vi "sub_main_imu.vi"(8 "error in":errorcluster) -> (0 "error out":errorcluster)   [LabVIEW 2019]
uses:
  Ctrl/gps-databuf.ctl
panel:
  out "n1":i32
  out "n":i32
  out "n2":i32
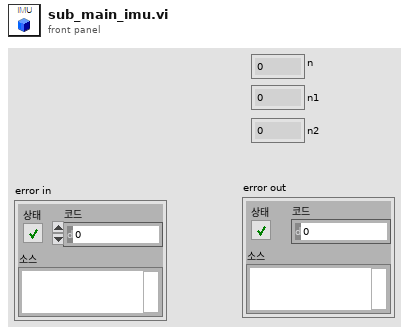
[diagram p1: front panel]
types:
  T1 = typedef "gps-databuf.ctl" = enum16{"read", "write"}
  T2 = typedef "imu-cfg.ctl" = cluster{"Port":refnum<visa-resource-name>, "offset":dbl, "rate":u32}
  T3 = cluster{"rawdata":string, "GPS Data":cluster{"Latitude":cluster{"Valid?":bool, "Latitude (Deg)":dbl}, "Longitude":cluster{"Valid?":bool, "Longitude (Deg)":dbl}, "Height":cluster{"Valid?":bool, "Height (m)":dbl}, "Undulation":cluster{"Valid?":bool, "Undulation(m)":dbl}, "North Vel":cluster{"Valid?":bool, "North Vel (m/s)":dbl}, "East Vel":cluster{"Valid?":bool, "East Vel (m/s)":dbl}, "Up Vel":cluster{"Valid?":bool, "Up Vel (m/s)":dbl}, "Roll":cluster{"Valid?":bool, "Roll (degrees)":dbl}, "Pitch":cluster{"Valid?":bool, "Pitch (degrees)":dbl}, "Azimuth":cluster{"Valid?":bool, "Azimuth (degrees)":dbl}, "Lat deviation":cluster{"Valid?":bool, "Lat deviation (m)":dbl}, "Long deviation":cluster{"Valid?":bool, "Long deviation (m)":dbl}, "Height deviation":cluster{"Valid?":bool, "Height deviation (m)":dbl}, "North vel deviation":cluster{"Valid?":bool, "North vel deviation (m/s)":dbl}, "East vel deviation":cluster{"Valid?":bool, "East vel deviation (m/s)":dbl}, "Up vel deviation":cluster{"Valid?":bool, "Up vel deviation (m/s)":dbl}, "Roll deviation":cluster{"Valid?":bool, "Roll deviation (degrees)":dbl}, "Pitch deviation":cluster{"Valid?":bool, "Pitch deviation (degrees)":dbl}, "Azimuth deviation":cluster{"Valid?":bool, "Azimuth deviation (degrees)":dbl}, "Ext sol status":cluster{"Valid?":bool, "Ext sol status":dbl}}, "Heading":dbl, "utm-1":cluster{"XN":dbl, "YE":dbl}}
  T4 = typedef "error_cluster.ctl" = cluster{"AGV":u8, "AGV Estop":u8, "Obstacle":u8, "Heading":u8, "Waypt":u8, "GNSS":u8, "VLP16":u8, "Cam":u8, "RPLidar":u8, "Joystick":u8, "IMU":u8}
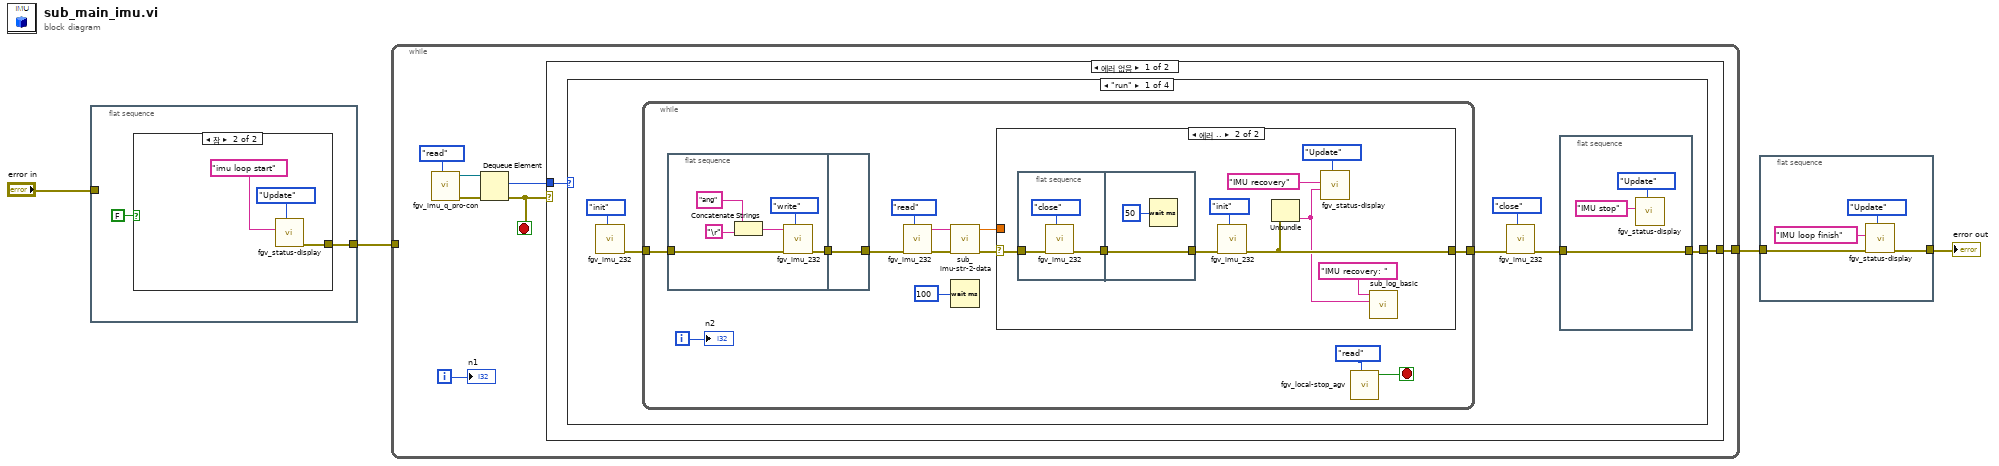
[diagram p0: block diagram]
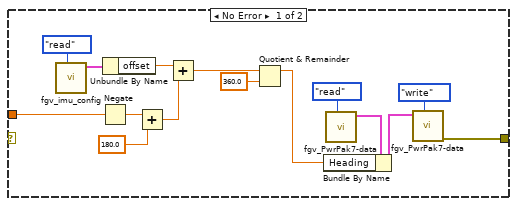
[diagram p2: hidden frame]
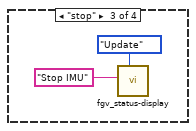
[diagram p4: hidden frame]
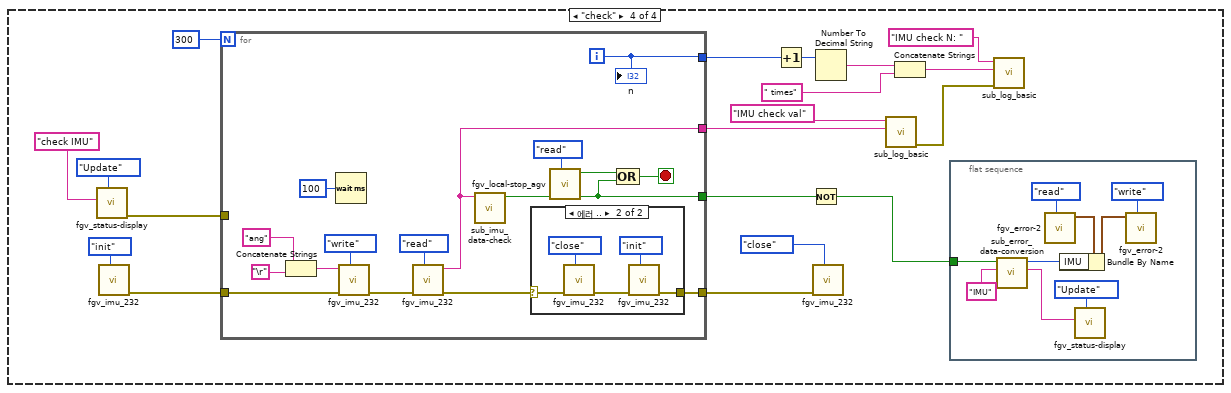
[diagram p5: hidden frame]
diagram:
  n1 = flat-sequence {
    tunnel: [w6] -> w3
    tunnel: "error in" -> [_]
    frame #0 {
      n2 = case shown="참" FALSE {
        tunnel: [_ w7] -> w6
        frame False {
        }
        frame True {
          n3 = call "fgv_status-display.vi"("Mode"=enum16{"Initial", "Update", "Clear"}."Update", "title"="imu loop start" ("String in 1")) -> ("error out"=w7:errorcluster)  [unwired: 9 in]
        }
      }
    }
  }
  n4 = while {
    tunnel: [w15] -> w1
    tunnel: w3 -> [_]
    i -> [w14]
    stop <- w13 stop-if-true
    n5 = call "fgv_imu_q_pro-con.vi"("cmd"=enum16{"create", "write", "read", "close"}."read") -> ("error out"=w10:errorcluster, "queue out"=w11:refnum<queue>)  [unwired: 9 in]
    n6 = Dequeue Element(queue=w11, error in (no error)=w10) -> (element=w16:enum16{"run", "check", "stop"}, error out=w13:errorcluster)  [unwired: 1 in, 2 out]
    n7 = case shown="에러 없음" w13 {
      tunnel: w16 -> [w18 _]
      tunnel: [w17 _] -> w15
      frame No Error {
        n8 = case shown="\"run\"" w18 {
          tunnel: [w24 _ _ _] -> w17
          frame "run" {
            n9 = call "fgv_imu_232.vi"("cmd"=enum16{"init", "read", "write", "close"}."init") -> ("error out"=w22:errorcluster)  [unwired: 8 in, 2 out]
            n10 = while {
              tunnel: [w37] -> w20
              tunnel: w22 -> [w35]
              i -> [w36]
              stop <- w39 stop-if-true
              n11 = flat-sequence {
                tunnel: w35 -> [w42]
                tunnel: [w41] -> w30
                tunnel: [w47] -> w34
                tunnel: w30 -> [w47]
                frame #0 {
                  n12 = Concatenate Strings("ang" ("문자열"), "\r") -> (w46:string)
                  n13 = call "fgv_imu_232.vi"("cmd"=enum16{"init", "read", "write", "close"}."write", "error in"=w42, "write buff"=w46) -> ("error out"=w41:errorcluster)  [unwired: 6 in, 2 out]
                }
                frame #1 {
                }
              }
              n14 = call "fgv_imu_232.vi"("cmd"=enum16{"init", "read", "write", "close"}."read", "error in"=w34) -> ("error out"=w32:errorcluster, "read_buffer"=w33:string)  [unwired: 7 in, 1 out]
              n15 = call "sub_imu-str-2-data.vi"("error in"=w32, "read buffer"=w33) -> ("error out"=w31:errorcluster, "yaw"=w29:dbl)  [unwired: 8 in]
              n16 = Wait (ms)(milliseconds to wait=u32 100 ("대기 시간 (ms)")) -> ()  [unwired: 1 out]
              n17 = case shown="에러 .." w31 {
                selector: w31 -> [_ w71]
                tunnel: [w57 w66] -> w37
                tunnel: w29 -> [w56 _]
                frame No Error {
                  n18 = call "fgv_imu_config.vi"("cmd"=enum16{"read", "write"}."read") -> ("IMU cfg out"=w53:T2)  [unwired: 9 in, 1 out]
                  n19 = Negate(x=w56) -> (-x=w55:dbl)
                  n20 = Unbundle By Name(w53) -> ("offset"=w52:dbl)
                  n21 = Add(x=w55, y=180.0) -> (x+y=w51:dbl)
                  n22 = Add(x=w52, y=w51) -> (x+y=w50:dbl)
                  n23 = Quotient & Remainder(x=w50, y=360.0) -> (x-y*floor(x/y)=w48:dbl)  [unwired: 1 out]
                  n24 = call "fgv_PwrPak7-data.vi"("cmd"=gps-databuf."read") -> ("data cluster out"=w59:T3)  [unwired: 9 in, 1 out]
                  n25 = Bundle By Name(cluster=w59, "Heading"=w48) -> (w60:T3)
                  n26 = call "fgv_PwrPak7-data.vi"("cmd"=gps-databuf."write", "data cluster in"=w60) -> ("error out"=w57:errorcluster)  [unwired: 8 in, 1 out]
                }
                frame Error {
                  n27 = flat-sequence {
                    tunnel: w71 -> [w73]
                    tunnel: [w72] -> w65
                    tunnel: [w76] -> w67
                    tunnel: w65 -> [w76]
                    frame #0 {
                      n28 = call "fgv_imu_232.vi"("cmd"=enum16{"init", "read", "write", "close"}."close", "error in"=w73) -> ("error out"=w72:errorcluster)  [unwired: 7 in, 2 out]
                    }
                    frame #1 {
                      n29 = Wait (ms)(milliseconds to wait=u32 50 ("대기 시간 (ms)")) -> ()  [unwired: 1 out]
                    }
                  }
                  n30 = call "fgv_imu_232.vi"("cmd"=enum16{"init", "read", "write", "close"}."init", "error in"=w67) -> ("error out"=w66:errorcluster)  [unwired: 7 in, 2 out]
                  n31 = Unbundle(w66) -> ("source"=w63:string)  [unwired: 2 out]
                  n32 = call "fgv_status-display.vi"("Mode"=enum16{"Initial", "Update", "Clear"}."Update", "detail"=w63, "title"="IMU recovery" ("String in 1")) -> ()  [unwired: 8 in, 1 out]
                  n33 = call "sub_log_basic.vi"("desc"=w63, "Title"="IMU recovery: ") -> ()  [unwired: 9 in, 1 out]
                }
              }
              n34 = call "fgv_local-stop_agv.vi"("cmd"=enum16{"ini", "read", "stop"}."read") -> ("stop status"=w39:bool)  [unwired: 10 in]
              "n2" <- w36
            }
            n35 = call "fgv_imu_232.vi"("cmd"=enum16{"init", "read", "write", "close"}."close", "error in"=w20) -> ("error out"=w19:errorcluster)  [unwired: 7 in, 2 out]
            n36 = flat-sequence {
              tunnel: [w25] -> w24
              tunnel: w19 -> [w25]
              frame #0 {
                n37 = call "fgv_status-display.vi"("Mode"=enum16{"Initial", "Update", "Clear"}."Update", "title"="IMU stop" ("String in 1")) -> ()  [unwired: 9 in, 1 out]
              }
            }
          }
          frame Default {
          }
          frame "stop" {
            n38 = call "fgv_status-display.vi"("Mode"=enum16{"Initial", "Update", "Clear"}."Update", "title"="Stop IMU" ("String in")) -> ()  [unwired: 9 in, 1 out]
          }
          frame "check" {
            n39 = call "fgv_status-display.vi"("Mode"=enum16{"Initial", "Update", "Clear"}."Update", "title"="check IMU" ("String in")) -> ("error out"=w79:errorcluster)  [unwired: 9 in]
            n40 = call "fgv_imu_232.vi"("cmd"=enum16{"init", "read", "write", "close"}."init") -> ("error out"=w93:errorcluster)  [unwired: 8 in, 2 out]
            n41 = for {
              N: 300 -> [_]
              tunnel: w93 -> [w113]
              tunnel: [w115] -> w91
              tunnel: [w107] -> w90
              tunnel: [w117] -> w86
              tunnel: [w108] -> w85
              tunnel: w79 -> [_]
              i -> [w117]
              stop <- w118 stop-if-true
              n42 = Concatenate Strings("ang" ("문자열"), "\r") -> (w111:string)
              n43 = Wait (ms)(milliseconds to wait=u32 100 ("대기 시간 (ms)")) -> ()  [unwired: 1 out]
              n44 = call "fgv_imu_232.vi"("cmd"=enum16{"init", "read", "write", "close"}."write", "error in"=w113, "write buff"=w111) -> ("error out"=w112:errorcluster)  [unwired: 6 in, 2 out]
              n45 = call "fgv_imu_232.vi"("cmd"=enum16{"init", "read", "write", "close"}."read", "error in"=w112) -> ("error out"=w116:errorcluster, "read_buffer"=w108:string)  [unwired: 7 in, 1 out]
              n46 = call "sub_imu_data-check.vi"("str"=w108) -> ("val"=w107:bool)  [unwired: 10 in]
              n47 = case shown="에러 .." w116 {
                selector: w116 -> [w123 w127]
                tunnel: [w123 w125] -> w115
                frame No Error {
                }
                frame Error {
                  n48 = call "fgv_imu_232.vi"("cmd"=enum16{"init", "read", "write", "close"}."close", "error in"=w127) -> ("error out"=w124:errorcluster)  [unwired: 7 in, 2 out]
                  n49 = call "fgv_imu_232.vi"("cmd"=enum16{"init", "read", "write", "close"}."init", "error in"=w124) -> ("error out"=w125:errorcluster)  [unwired: 7 in, 2 out]
                }
              }
              n50 = call "fgv_local-stop_agv.vi"("cmd"=enum16{"ini", "read", "stop"}."read") -> ("stop status"=w119:bool)  [unwired: 10 in]
              n51 = Compound Arithmetic op=OR ("복합 연산")(w119, w107) -> (w118:bool)
              "n" <- w117
            }
            n52 = Increment(x=w86) -> (x+1=w89:i32)
            n53 = Not(x=w90) -> (.not. x?=w80:bool)
            n54 = call "fgv_imu_232.vi"("cmd"=enum16{"init", "read", "write", "close"}."close", "error in"=w91) -> ()  [unwired: 7 in, 3 out]
            n55 = Number To Decimal String(number=w89) -> (decimal integer string=w88:string)  [unwired: 1 in]
            n56 = call "sub_log_basic.vi"("desc"=w85, "Title"="IMU check val") -> ("error out"=w81:errorcluster)  [unwired: 9 in]
            n57 = Concatenate Strings(w88, " times" ("문자열")) -> (w83:string)
            n58 = flat-sequence {
              tunnel: w80 -> [w101]
              frame #0 {
                n59 = call "sub_error_data-conversion.vi"("name"="IMU", "error status"=w101) -> ("check result string"=w98:string, "error conversion out"=w106:u8)  [unwired: 8 in]
                n60 = call "fgv_error-2.vi"("cmd"=enum16{"init", "read", "write"}."read") -> ("Error cluster out"=w105:T4)  [unwired: 9 in, 1 out]
                n61 = Bundle By Name(cluster=w105, "IMU"=w106) -> (w104:T4)
                n62 = call "fgv_status-display.vi"("Mode"=enum16{"Initial", "Update", "Clear"}."Update", "title"=w98) -> ()  [unwired: 9 in, 1 out]
                n63 = call "fgv_error-2.vi"("cmd"=enum16{"init", "read", "write"}."write", "Error cluster"=w104) -> ()  [unwired: 8 in, 2 out]
              }
            }
            n64 = call "sub_log_basic.vi"("error in"=w81, "desc"=w83, "Title"="IMU check N: ") -> ()  [unwired: 8 in, 1 out]
          }
        }
      }
      frame Error {
      }
    }
    "n1" <- w14
  }
  n65 = flat-sequence {
    tunnel: [w130] -> w2
    tunnel: w1 -> [w129]
    frame #0 {
      n66 = call "fgv_status-display.vi"("Mode"=enum16{"Initial", "Update", "Clear"}."Update", "error in"=w129, "title"="IMU loop finish" ("String in 1")) -> ("error out"=w130:errorcluster)  [unwired: 8 in]
    }
  }
  "error out" <- w2
